vi "文件夹编号.vi"(7 "模式":enum16{"读", "写", "读写"}(ring), 8 "error in (no error)":errorcluster caption="错误输入（无错误）", 10 "文件夹序号in":u32, 11 "设置文件路径":path) -> (0 "error out":errorcluster caption="错误输出", 2 "文件夹序号out":u32)   [LabVIEW 2018]
uses:
  <vilib>/Utility/config.llb/Read Key (U32).vi
  <vilib>/Utility/config.llb/Write Key (U32).vi
  <vilib>/Utility/config.llb/NI_LVConfig.lvlib
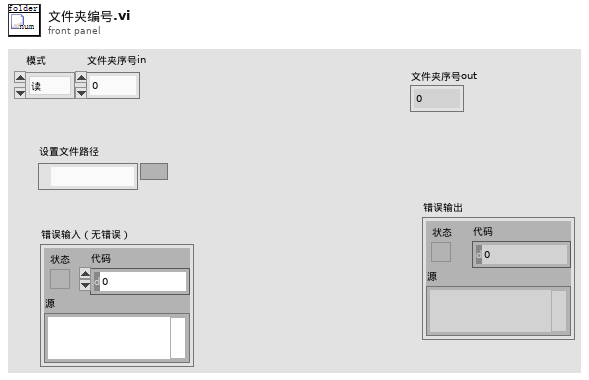
[diagram p1: front panel]
types:
  T1 = typedef "NI_LVConfig.lvlib/Config Data RefNum.ctl" = refnum<k1>
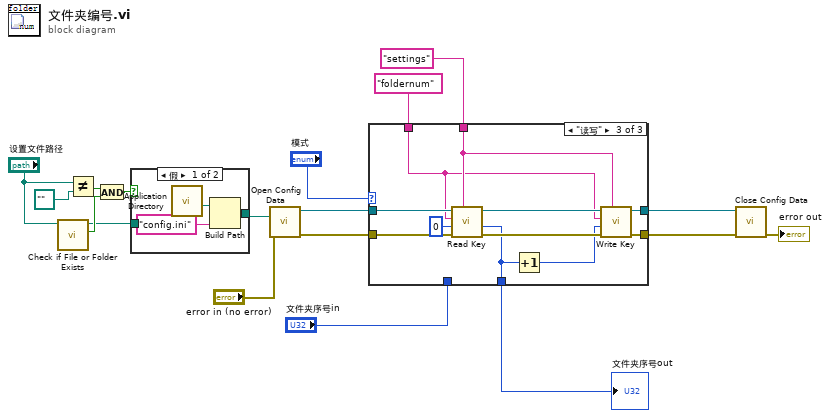
[diagram p0: block diagram]
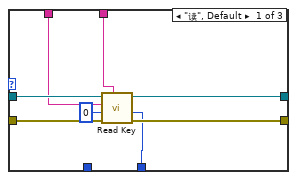
[diagram p2: hidden frame]
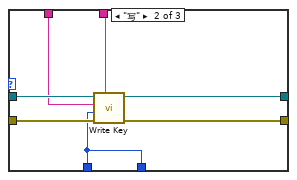
[diagram p3: hidden frame]
diagram:
  n1 = call <vilib>:"Check if File or Folder Exists.vi"("path"="设置文件路径") -> ("file or folder exists?"=w12:bool, "dup path"=w10:path)  [unwired: 8 in, 1 out]
  n2 = Not Equal?(x="设置文件路径", y=path "" ("添加的路径")) -> (x != y?=w13:bool)
  n3 = And(x=w13, y=w12) -> (x .and. y?=w11:bool)
  n4 = case shown="假" w11 {
    tunnel: [w19 w22] -> w16
    tunnel: w10 -> [_ w22]
    frame False {
      n5 = call <vilib>:"Application Directory.vi"() -> ("Application Directory"=w21:path)
      n6 = Build Path(base path=w21, name or relative path="config.ini" ("名称或相对路径")) -> (appended path=w19:path)
    }
    frame True {
    }
  }
  n7 = call <vilib>:"Open Config Data.vi"("error in (no error)"="error in (no error)", "configuration file path"=w16) -> ("error out"=w7:errorcluster, "refnum"=w9:T1)  [unwired: 7 in, 1 out]
  n8 = case shown="\"读写\"" "模式" {
    tunnel: w9 -> [w30 w37 w48]
    tunnel: [w29 w35 w46] -> w8
    tunnel: w7 -> [w28 w36 w45]
    tunnel: [w27 w34 w43] -> w6
    tunnel: [w23 w31 w41] -> w5
    tunnel: "settings" ("section") -> [w26 w33 w39]
    tunnel: "foldernum" -> [w25 w32 w38]
    tunnel: "文件夹序号in" -> [_ w31 _]
    frame "读", Default {
      n9 = call-poly <vilib>:"Read Key.vi"("section"=w26, "error in (no error)"=w28, "default value"=u32 0, "key"=w25, "refnum"=w30) -> ("error out"=w27:errorcluster, "value"=w23:u32, "refnum out"=w29:T1)  [unwired: 3 in, 1 out]
    }
    frame "写" {
      n10 = call-poly <vilib>:"Write Key.vi"("section"=w33, "error in (no error)"=w36, "value"=w31, "key"=w32, "refnum"=w37) -> ("error out"=w34:errorcluster, "refnum out"=w35:T1)  [unwired: 4 in, 1 out]
    }
    frame "读写" {
      n11 = call-poly <vilib>:"Read Key.vi"("section"=w39, "error in (no error)"=w45, "default value"=u32 0, "key"=w38, "refnum"=w48) -> ("error out"=w44:errorcluster, "value"=w41:u32, "refnum out"=w47:T1)  [unwired: 3 in, 1 out]
      n12 = Increment(x=w41) -> (x+1=w40:u32)
      n13 = call-poly <vilib>:"Write Key.vi"("section"=w39, "error in (no error)"=w44, "value"=w40, "key"=w38, "refnum"=w47) -> ("error out"=w43:errorcluster, "refnum out"=w46:T1)  [unwired: 4 in, 1 out]
    }
  }
  "文件夹序号out" <- w5
  n14 = call <vilib>:"Close Config Data.vi"("error in (no error)"=w6, "refnum"=w8) -> ("error out"=→"error out":errorcluster)  [unwired: 8 in, 1 out]
